vi "SetValueByItemTagArray.vi"(0 "VI Reference In":refnum<vi>, 2 "delimiter (>>)":string=">>", 5 "Control Path":string, 7 "Item Tags Array":string[](array[string]), 11 "Error In":errorcluster) -> (4 "VI Reference Out":refnum<vi>, 15 "Error Out":errorcluster)   [LabVIEW 2016, in "Drona.lvlib" / "ControlValue.lvlib" / "StimulusTree.lvlib"]
doc: "Sets value(signaling) for the multi-select tree control whose item tags are specified as an array. \n\nThe input control name is given as a string , incase of path, use delimiters inbetween the path."
uses:
  StimulusTree.lvlib
  <vilib>/Utility/error.llb/Error Cluster From Error Code.vi
  <vilib>/ErrorRing/Error Ring.xnode
  Drona.lvlib
  Get/GetControlRef/GetControlRef.lvlib
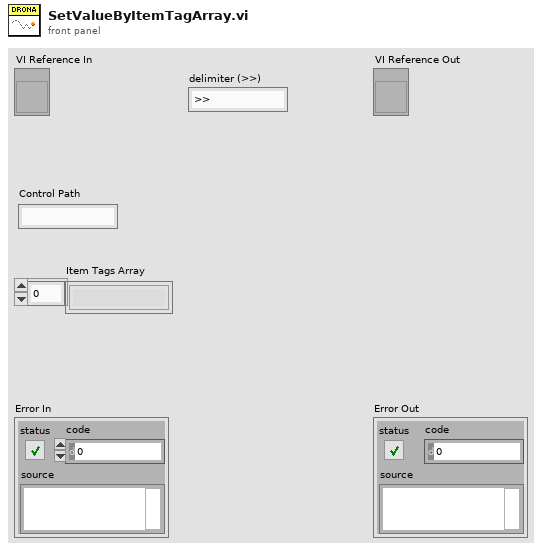
[diagram p1: front panel]
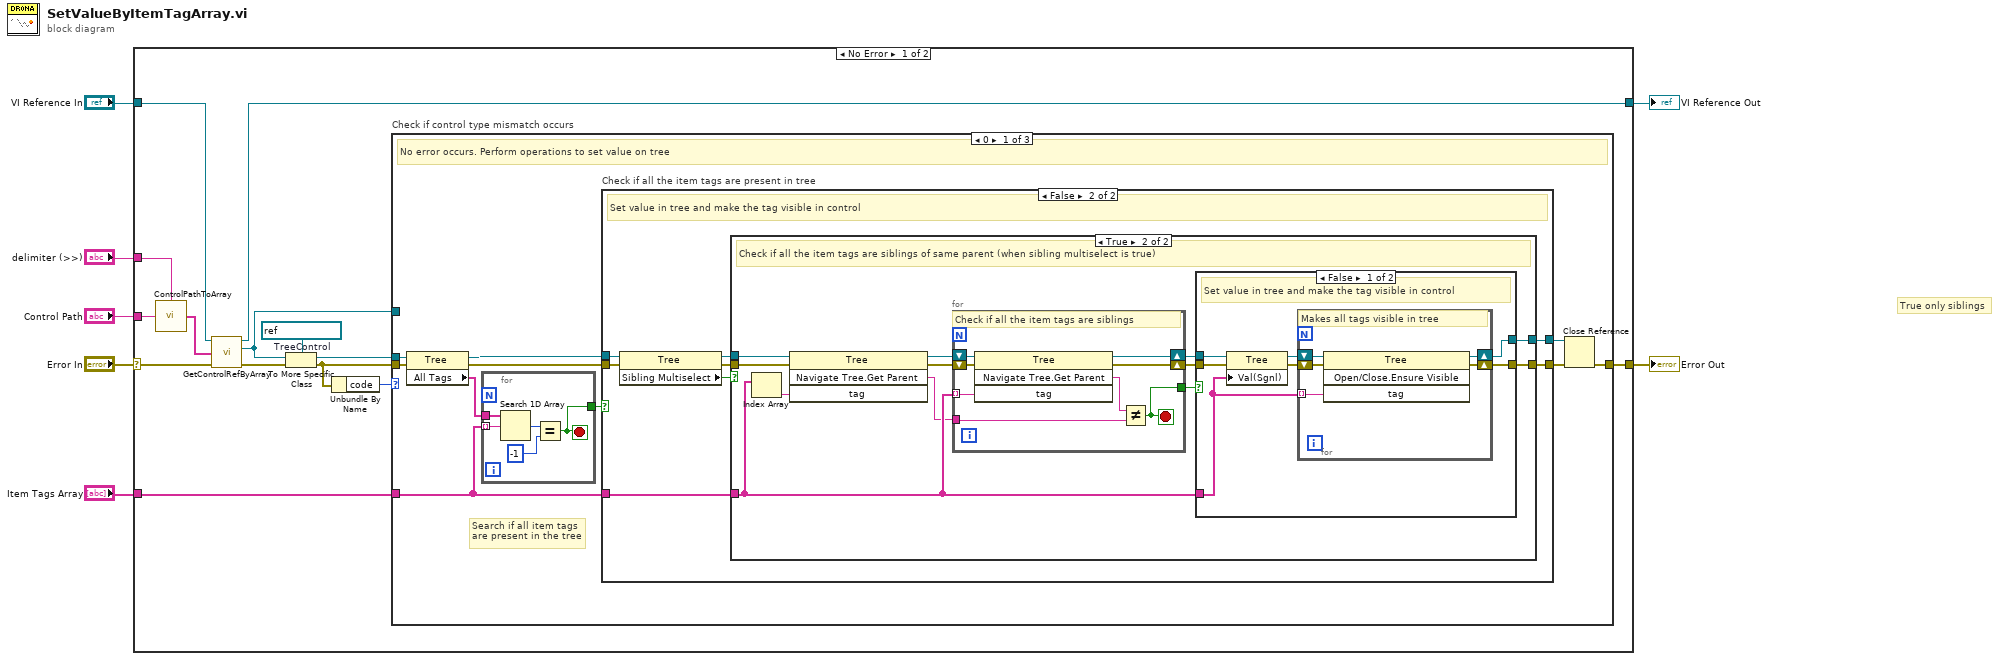
[diagram p0: block diagram]
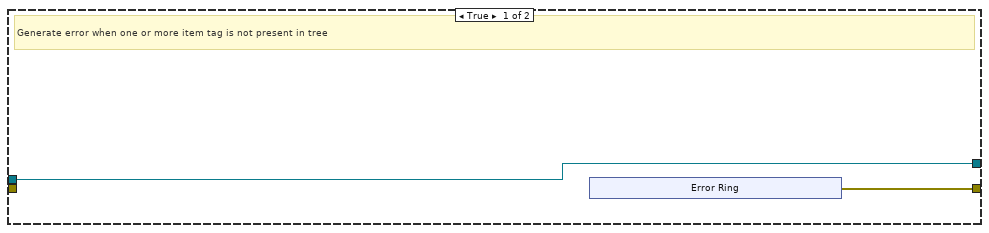
[diagram p2: hidden frame]
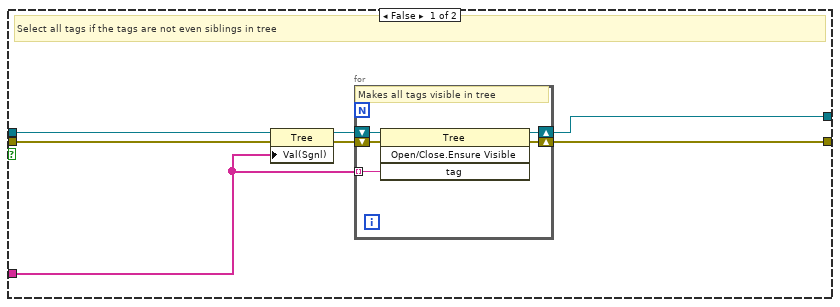
[diagram p3: hidden frame]
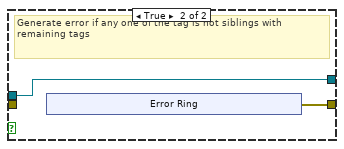
[diagram p4: hidden frame]
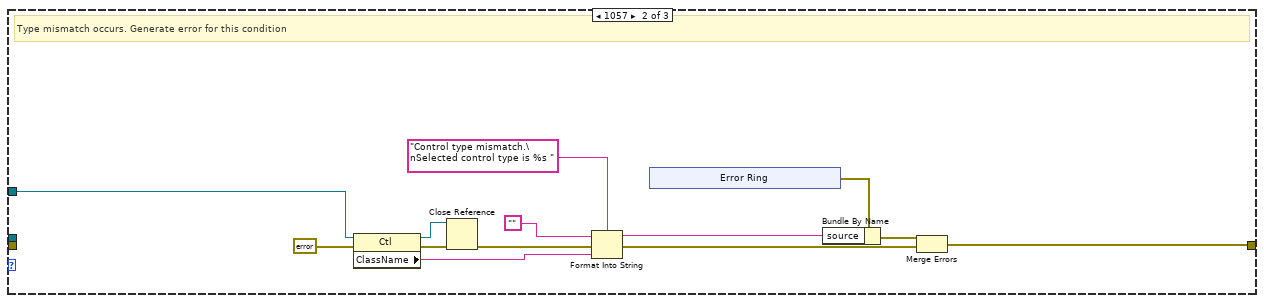
[diagram p5: hidden frame]
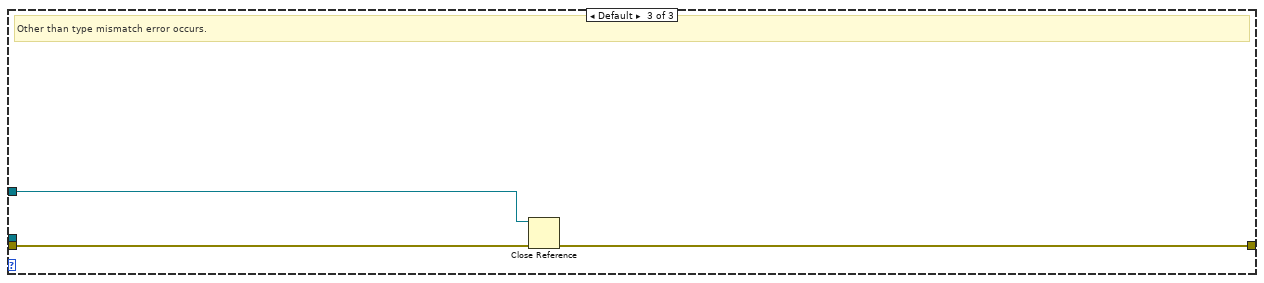
[diagram p6: hidden frame]
diagram:
  # "True only siblings"
  n1 = case shown="No Error" "Error In" {
    selector: "Error In" -> [w18 w125]
    tunnel: [w8 w125] -> w6
    tunnel: "VI Reference In" -> [w17 w124]
    tunnel: "Control Path" -> [w20 _]
    tunnel: [w14 w124] -> w3
    tunnel: "delimiter (>>)" -> [w19 _]
    tunnel: "Item Tags Array" -> [w13 _]
    frame No Error {
      w21 = refnum<vi> refnum  # TreeControl
      n2 = call "ControlPathToArray.vi"("Control Name"=w20, "delimiter (>>)"=w19) -> ("Control Path"=w16:string[])
      n3 = call "GetControlRefByArray.vi"("VI Reference In"=w17, "Control Path"=w16, "error In"=w18) -> ("VI Reference Out"=w14:refnum<vi>, "Ctl Refnum"=w10:refnum<vi>, "error out"=w15:errorcluster)  [unwired: 10 in]
      n4 = To More Specific Class(target class=w21, reference=w10, error in=w15) -> (specific class reference=w11:refnum<vi>, error out=w12:errorcluster)
      n5 = Unbundle By Name(w12) -> ("code"=w9:i32)
      n6 = case "Check if control type mismatch occurs" shown="0" w9 {
        tunnel: [w31 w105 w122] -> w8
        tunnel: w11 -> [w26 _ _]
        tunnel: w13 -> [w23 _ _]
        tunnel: w10 -> [_ w115 w121]
        tunnel: w12 -> [w30 _ w123]
        frame 0 {
          # "Search if all item tags \nare present in the tree"
          # "No error occurs. Perform operations to set value on tree"
          n7 = property class="Tree"(reference=w26, error in=w30) -> (reference out=w25:refnum<vi>, error out=w27:errorcluster, "All Tags"=w24:string[])
          n8 = for {
            tunnel: w24 -> [w36]
            tunnel: w23 -> [w35] mode=indexing
            tunnel: [w32] -> w22
            stop <- w32 stop-if-true
            n9 = Search 1D Array(1D array=w36, element=w35) -> (index of element=w34:i32)  [unwired: 1 in]
            n10 = Equal?(x=w34, y=-1) -> (x = y?=w32:bool)
          }
          n11 = case "Check if all the item tags are present in tree" shown="False" w22 {
            tunnel: [w37 w50] -> w29
            tunnel: [w38 w49] -> w28
            tunnel: w27 -> [_ w51]
            tunnel: w25 -> [w38 w46]
            tunnel: w23 -> [_ w48]
            frame True {
              # "Generate error when one or more item tag is not present in tree"
              n12 = xnode "Error Ring"() -> ("error out"=w37:errorcluster)
            }
            frame False {
              # "Set value in tree and make the tag visible in control"
              n13 = property class="Tree"(reference=w46, error in=w51) -> (reference out=w44:refnum<vi>, error out=w47:errorcluster, "Sibling Multiselect"=w45:bool)
              n14 = case shown="True" w45 {
                tunnel: [w57 w75] -> w50
                tunnel: [w55 w74] -> w49
                tunnel: w48 -> [w54 w70]
                tunnel: w47 -> [w53 w73]
                tunnel: w44 -> [w52 w71]
                frame False {
                  # "Select all tags if the tags are not even siblings in tree"
                  n15 = property class="Tree"(reference=w52, error in=w53, "Val(Sgnl)"=w54) -> (reference out=w56:refnum<vi>, error out=w58:errorcluster)
                  n16 = for {
                    shift-right: [w62] -> w57
                    shift-left: w58 -> [w63]
                    shift-right: [w60] -> w55
                    shift-left: w56 -> [w61]
                    tunnel: w54 -> [w59] mode=indexing
                    # "Makes all tags visible in tree"
                    n17 = invoke class="Tree" method="Open/Close.Ensure Visible"(reference=w61, error in=w63, "tag"=w59) -> (reference out=w60:refnum<vi>, error out=w62:errorcluster)  [unwired: 1 in, 2 out]
                  }
                }
                frame True {
                  # "Check if all the item tags are siblings of same parent (when sibling multiselect is true)"
                  n18 = Index Array(array=w70) -> (element=w69:string)  [unwired: 1 in]
                  n19 = invoke class="Tree" method="Navigate Tree.Get Parent"(reference=w71, error in=w73, "tag"=w69) -> (reference out=w64:refnum<vi>, error out=w72:errorcluster, "Navigate Tree:Get Parent"=w68:string)  [unwired: 1 in, 1 out]
                  n20 = for {
                    tunnel: w70 -> [w100] mode=indexing
                    shift-right: [w98] -> w66
                    shift-left: w72 -> [w101]
                    shift-right: [w99] -> w65
                    shift-left: w64 -> [w102]
                    tunnel: w68 -> [w96]
                    tunnel: [w95] -> w67
                    stop <- w95 stop-if-true
                    # "Check if all the item tags are siblings"
                    n21 = invoke class="Tree" method="Navigate Tree.Get Parent"(reference=w102, error in=w101, "tag"=w100) -> (reference out=w99:refnum<vi>, error out=w98:errorcluster, "Navigate Tree:Get Parent"=w97:string)  [unwired: 1 in, 1 out]
                    n22 = Not Equal?(x=w97, y=w96) -> (x != y?=w95:bool)
                  }
                  n23 = case shown="False" w67 {
                    tunnel: [w81 w88] -> w75
                    tunnel: [w79 w89] -> w74
                    tunnel: w70 -> [w78 _]
                    tunnel: w66 -> [w77 _]
                    tunnel: w65 -> [w76 w89]
                    frame False {
                      # "Set value in tree and make the tag visible in control"
                      n24 = property class="Tree"(reference=w76, error in=w77, "Val(Sgnl)"=w78) -> (reference out=w80:refnum<vi>, error out=w82:errorcluster)
                      n25 = for {
                        shift-right: [w86] -> w81
                        shift-left: w82 -> [w87]
                        shift-right: [w84] -> w79
                        shift-left: w80 -> [w85]
                        tunnel: w78 -> [w83] mode=indexing
                        # "Makes all tags visible in tree"
                        n26 = invoke class="Tree" method="Open/Close.Ensure Visible"(reference=w85, error in=w87, "tag"=w83) -> (reference out=w84:refnum<vi>, error out=w86:errorcluster)  [unwired: 1 in, 2 out]
                      }
                    }
                    frame True {
                      # "Generate error if any one of the tag is not siblings with remaining tags"
                      n27 = xnode "Error Ring"() -> ("error out"=w88:errorcluster)
                    }
                  }
                }
              }
            }
          }
          n28 = Close Reference(reference=w28, error in (no error)=w29) -> (error out=w31:errorcluster)
        }
        frame 1057 {
          # "Type mismatch occurs. Generate error for this condition"
          n29 = property class="Ctl"(reference=w115, error in=errorcluster {"status"=FALSE, "code"=0, "source"=""} ("error out")) -> (reference out=w103:refnum<vi>, error out=w114:errorcluster, "ClassName"=w111:string)
          n30 = Close Reference(reference=w103, error in (no error)=w114) -> (error out=w104:errorcluster)
          n31 = Format Into String(format string="Control type mismatch.\nSelected control type is %s ", initial string="", error in=w104, w111) -> (resulting string=w108:string, error out=w106:errorcluster)
          n32 = xnode "Error Ring"() -> ("error out"=w109:errorcluster)
          n33 = Bundle By Name(cluster=w109, "source"=w108) -> (w107:errorcluster)
          n34 = Merge Errors(w107, w106) -> (w105:errorcluster)
        }
        frame Default {
          # "Other than type mismatch error occurs."
          n35 = Close Reference(reference=w121, error in (no error)=w123) -> (error out=w122:errorcluster)
        }
      }
    }
    frame Error {
    }
  }
  "Error Out" <- w6
  "VI Reference Out" <- w3
